vi "Publish Random Data.vi"(8 "error in":errorcluster, 10 "Dataset Length":i32=100, 11 "Variable References In":refnum<k21>[](array[refnum])) -> (0 "error out":errorcluster, 3 "Variable References Out":refnum<k21>[](array[refnum]))   [LabVIEW 2017, in "DTACQ - Network Enabled Device Driver.lvlib"]
uses:
  DTACQ - Network Enabled Device Driver.lvlib
  Network Shared Variables/Typedefs/X and Y Variant Arrays--Cluster.ctl
  Network Shared Variables/Shared Variables Library.lvlib
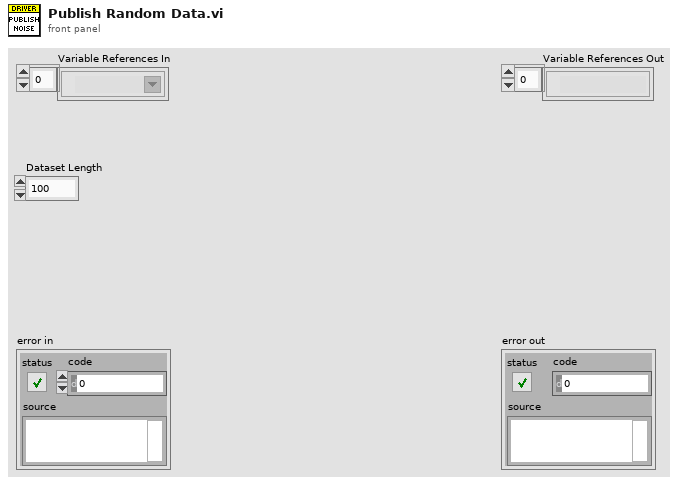
[diagram p1: front panel]
types:
  T1 = typedef "Shared Variables Library.lvlib/X and Y Variant Arrays--Cluster.ctl" = cluster{"X-Data":variant[], "Y-Data":variant[]}
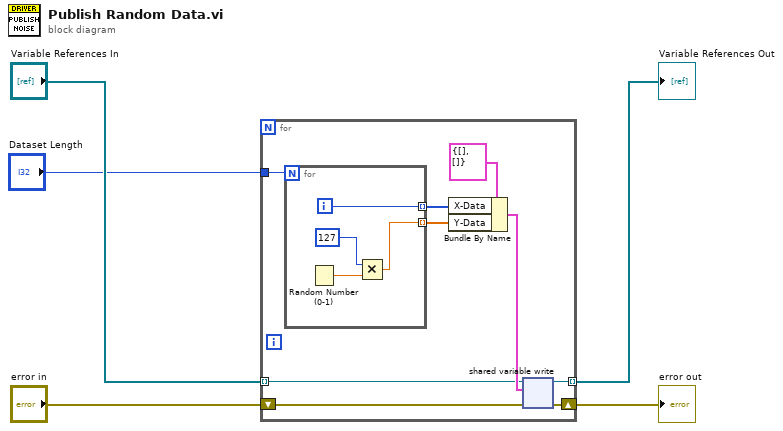
[diagram p0: block diagram]
diagram:
  n1 = for {
    tunnel: [w10] -> w4 mode=indexing
    shift-right: [w11] -> w3
    shift-left: "error in" -> [w12]
    tunnel: "Variable References In" -> [w9] mode=indexing
    tunnel: "Dataset Length" -> [w8]
    n2 = for {
      N: w8 -> [_]
      tunnel: [w18] -> w7 mode=indexing
      tunnel: [w15] -> w6 mode=indexing
      i -> [w18]
      n3 = Random Number (0-1)() -> (number: 0 to 1=w17:dbl)
      n4 = Multiply(x=i8 127, y=w17) -> (x*y=w15:dbl)
    }
    n5 = Bundle By Name(cluster=T1 {"X-Data"=[], "Y-Data"=[]} ("Data Cluster"), "X-Data"=w7, "Y-Data"=w6) -> (w13:T1)
    n6 = shared-variable-write(w9, w12, w13) -> (w10:refnum<k21>, w11:errorcluster)
  }
  "Variable References Out" <- w4
  "error out" <- w3
